vi "DLSATKdll.vi"(8 "error in (no error)":errorcluster, 11 "Inputs":cluster{"icomp":i32, "t":dbl}) -> (0 "error out":errorcluster, 3 "Outputs":T1)   [LabVIEW 2021]
doc: "subroutine DLSATKdll(icomp, t, D, ierr, herr, herr_length)\n\nCompute pure fluid saturated liquid density with appropriate equation.\nParameters\n\nINPUTS: \nicomp -- Component i\nt -- Temperature [K]\n\nOUTPUTS:\nD -- Saturated liquid density [mol/L]\nierr -- Error flag: 0 - Successful 1 - T>Tc -2 - D<Dc 501 - No equation available\nherr -- Error string \nherr_length -- length of variable herr (default: 255)"
uses:
  REFPROP.dll
panel:
  # "REFPROP-DLSATKdll.vi"
  # "void  DLSATKdll(int32_t *icomp, double *t, double *D, int32_t *ierr, CStr herr, int32_t ln)"
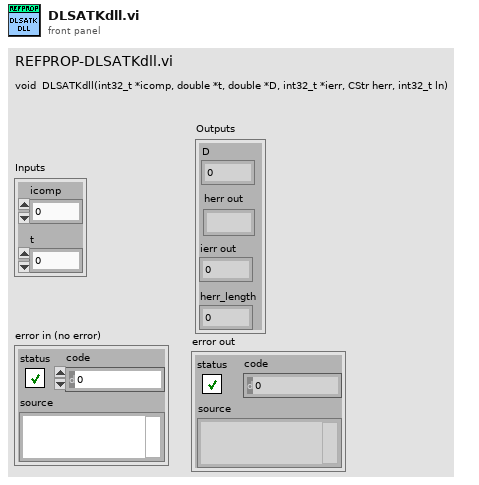
[diagram p1: front panel]
types:
  T1 = cluster{"D":dbl, "ierr out":i32, "herr out":string, "herr_length":i32}
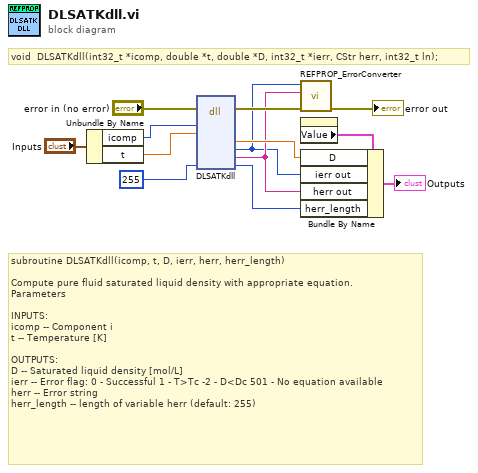
[diagram p0: block diagram]
diagram:
  # "void  DLSATKdll(int32_t *icomp, double *t, double *D, int32_t *ierr, CStr herr, int32_t ln);"
  # "subroutine DLSATKdll(icomp, t, D, ierr, herr, herr_length)\n\nCompute pure fluid saturated liquid density with appropriate equation.\nParameters\n\nINPUTS: \nicomp -- Component i\nt -- Temperature [K]\n\nOUTPUTS:\nD -- Saturated liquid density [mol/L]\nierr -- Error flag: 0 - Successful 1 - T>Tc -2 - D<Dc 501 - No equation available\nherr -- Error string \nherr_length -- length of variable herr (default: 255)"
  n1 = Unbundle By Name("Inputs") -> ("icomp"=w9:i32, "t"=w8:dbl)
  n2 = dll-call lib="C:/Users/lauria/OneDrive - National Institute of Standards and Technology (NIST)/LabVIEW Projects/7 REFPROP/REFPROP-wrappers-master/REFPROP-wrappers-master/wrappers/Labview/REFPROP/REFPROP.*" fn="DLSATKdll"(error in="error in (no error)", "icomp"=w9, "t"=w8, "herr_length"=255 ("ln")) -> (error out=w12:errorcluster, "D"=w5:dbl, "ierr"=w1:i32, "herr"=w2:string, "herr_length"=w4:i32)  [unwired: 8 in, 1 out]
  n3 = call "REFPROP_ErrorConverter.vi"("error in (no error)"=w12, "Error Message"=w2, "Error Code"=w1) -> ("error out"=→"error out":errorcluster)  [unwired: 8 in]
  n4 = property on="Outputs" class="Clust (strict)"() -> ("Value"=w6:T1)  [unwired: 2 in, 2 out]
  n5 = Bundle By Name(cluster=w6, "D"=w5, "ierr out"=w1, "herr out"=w2, "herr_length"=w4) -> (→"Outputs":T1)
